vi "Message.vi"(7 "Status":refnum<vi>, 10 "error in (no error)":errorcluster, 11 "Status":string) -> (2 "error out":errorcluster)   [LabVIEW 2019, in "VIPM.lvclass"]
uses:
  VIPM.lvclass
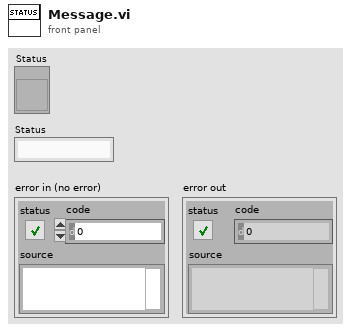
[diagram p1: front panel]
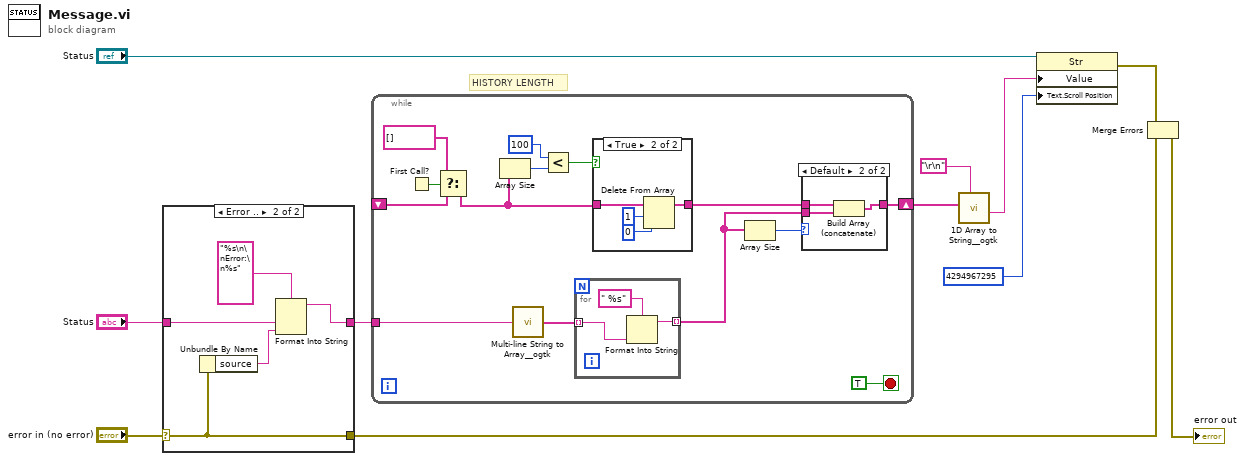
[diagram p0: block diagram]
diagram:
  # "HISTORY LENGTH"
  n1 = case shown="Error .." "error in (no error)" {
    selector: "error in (no error)" -> [w12 w14]
    tunnel: "Status" -> [w13 w15]
    tunnel: [w13 w17] -> w7
    tunnel: [w12 w14] -> w4
    frame No Error {
    }
    frame Error {
      n2 = Unbundle By Name(w14) -> ("source"=w16:string)
      n3 = Format Into String(format string="%s\n\nError:\n%s", w15, w16) -> (resulting string=w17:string)  [unwired: 2 in, 1 out]
    }
  }
  n4 = while {
    tunnel: w7 -> [w22]
    shift-right: [w29] -> w3
    shift-left: _ -> [w25]
    stop <- TRUE stop-if-true
    n5 = First Call?() -> (First Call?: T/F=w26:bool)
    n6 = Select(t=string[] [], s=w26, f=w25) -> (s? t:f=w24:string[])
    n7 = Array Size(array=w24) -> (size(s)=w31:i32)
    n8 = call <userlib>:"Multi-line String to Array__ogtk.vi"("string"=w22) -> ("lines"=w21:string[])
    n9 = Less?(x=100 ("length"), y=w31) -> (x < y?=w28:bool)
    n10 = for {
      tunnel: [w33] -> w20 mode=indexing
      tunnel: w21 -> [w34] mode=indexing
      n11 = Format Into String(format string=" %s", w34) -> (resulting string=w33:string)  [unwired: 2 in, 1 out]
    }
    n12 = case shown="True" w28 {
      tunnel: w24 -> [w36 w37]
      tunnel: [w36 w39] -> w32
      frame False {
      }
      frame True {
        n13 = Delete From Array(array=w37, length=1, index=0) -> (array with subset deleted=w39:string[])  [unwired: 1 out]
      }
    }
    n14 = Array Size(array=w20) -> (size(s)=w19:i32)
    n15 = case shown="Default" w19 {
      tunnel: w32 -> [w41 w42]
      tunnel: [w41 w44] -> w29
      tunnel: w20 -> [_ w43]
      frame 0 {
      }
      frame Default {
        n16 = Build Array (concatenate)(w42, w43) -> (w44:string[])
      }
    }
  }
  n17 = call <userlib>:"1D Array to String__ogtk.vi"("delimiter (Tab)"="\r\n", "Array of Strings"=w3) -> ("delimited string"=w1:string)  [unwired: 9 in]
  n18 = property class="Str"(reference="Status", "Value"=w1, "Text.Scroll Position"=u32 4294967295) -> (error out=w6:errorcluster)  [unwired: 1 in, 1 out]
  n19 = Merge Errors(w6, w4) -> (→"error out":errorcluster)
